vi "Get Obj by Type.vi"(8 "error in (no error)":errorcluster, 10 "Type":refnum<class "Analyze BaseClass.lvclass">, 11 "Analyze Compound Analysis Base in":refnum<class "Analyze Compound Analysis Base.lvclass">) -> (0 "error out":errorcluster, 1 "found?":bool, 2 "Analyze Obj":refnum<class "Analyze BaseClass.lvclass">, 3 "Analyze Compound Analysis Base out":refnum<class "Analyze Compound Analysis Base.lvclass">)   [LabVIEW 2014, in "Analyze.lvlib" / "Analyze Compound Analysis Base.lvclass"]
uses:
  Analyze Compound Analysis Base.lvclass
  Analyze BaseClass/Analyze BaseClass/Analyze BaseClass.lvclass
  Analyze Compound Analysis Base.lvclass/Analyze Compound Analysis Base.ctl
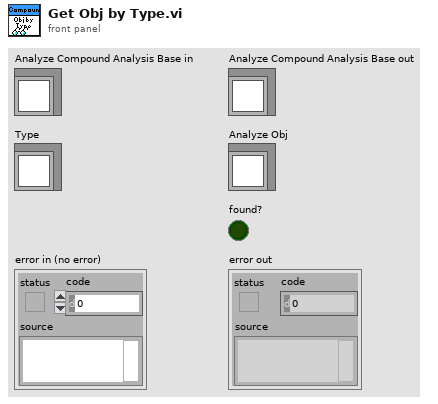
[diagram p1: front panel]
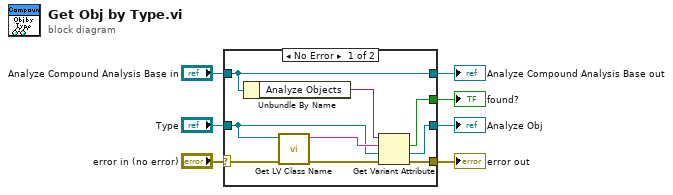
[diagram p0: block diagram]
diagram:
  n1 = case shown="No Error" "error in (no error)" {
    selector: "error in (no error)" -> [w10 w19]
    tunnel: [w8 w19] -> w5
    tunnel: [w16 w18] -> w4
    tunnel: "Analyze Compound Analysis Base in" -> [w16 w18]
    tunnel: "Type" -> [w13 w17]
    tunnel: [w12 w17] -> w2
    tunnel: [w11 _] -> w1
    frame No Error {
      n2 = Unbundle By Name(w16) -> ("Analyze Objects"=w15:variant)
      n3 = call <vilib>:"Get LV Class Name.vi"("error in (no error)"=w10, "object"=w13) -> ("error out"=w9:errorcluster, "class name"=w14:string)  [unwired: 8 in]
      n4 = Get Variant Attribute(Variant=w15, name=w14, default value (empty Variant)=w13, error in=w9) -> (found=w11:bool, value=w12:refnum<class "Analyze BaseClass.lvclass">, error out=w8:errorcluster)  [unwired: 1 out]
    }
    frame Error {
    }
  }
  "error out" <- w5
  "Analyze Compound Analysis Base out" <- w4
  "Analyze Obj" <- w2
  "found?" <- w1
